vi "Pid_v21.vi"() -> ()   [LabVIEW 2020]
doc: "This example demonstrates how to simulate a general PID controller."
uses:
  <vilib>/addons/control/pid/pid.llb/PID (DBL).vi
  <vilib>/addons/control/pid/NI_PID_pid.lvlib
panel:
  in  "r - Set point":dbl(slide)=4.965034965034965 scale=0.0..10.0
  out "y - Iesirea":dbl(slide)=0.4195804195804196 scale=0.0..10.0
  out "u":dbl(slide)=0.27972027972027974 scale=0.0..10.0
  out "U - comanda":dbl(graph)=4.96503496506626
  in  "PID gains":T1={"proportional gain (Kc)"=20.0, "integral time (Ti, min)"=0.008, "derivative time (Td, min)"=0.001} {"derivative time (Td, min)" format="%.3f"; "integral time (Ti, min)" format="%.3f"; "proportional gain (Kc)" format="%.3f"}
  in  "Stop":bool
  out "u,y,r":T2(graph)={"Plant Output"=4.96503496506626, "output"=4.965034965036714, "r - Set point"=4.965034965034965}
  # "Overview: This example demonstrates how to simulate a simple PID loop controller.\nInstructions:\n1. Run the VI and observe the Process variable (PV) following the Setpoint (SP) value while the output of the controller, also called Manipulated variable (MV), changes to keep both values near each other.\n2. After it settles down (value of PV and SP are near each other), change SP. You can just move the 'blue' arrow on the indicator. The MV will change to drive PV to SP again.\n3. Click Stop to stop the VI."
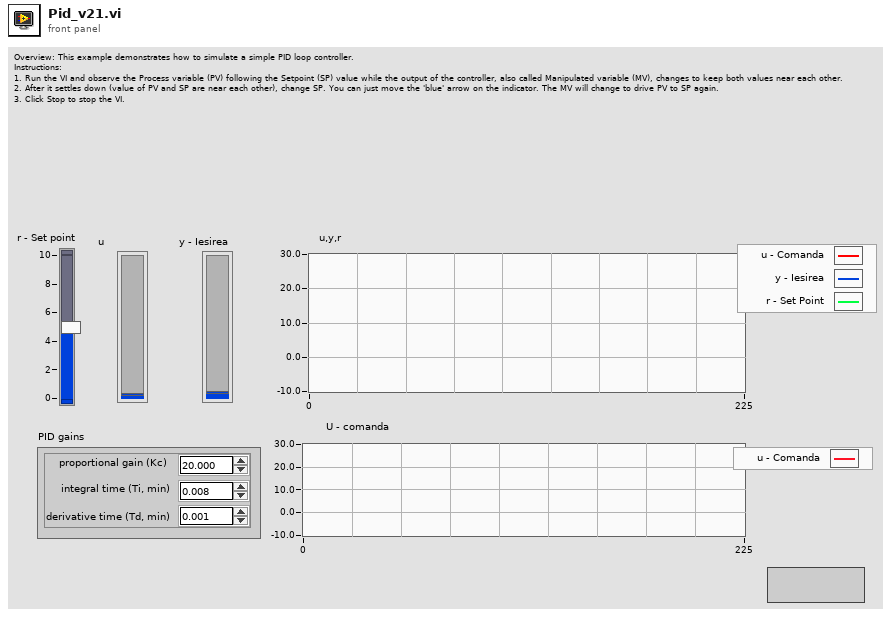
[diagram p1: front panel]
types:
  T1 = cluster{"proportional gain (Kc)":dbl, "integral time (Ti, min)":dbl, "derivative time (Td, min)":dbl}
  T2 = cluster{"Plant Output":dbl, "output":dbl, "r - Set point":dbl}
  T3 = cluster{"output":dbl, "y":dbl, "r - Set point":dbl}
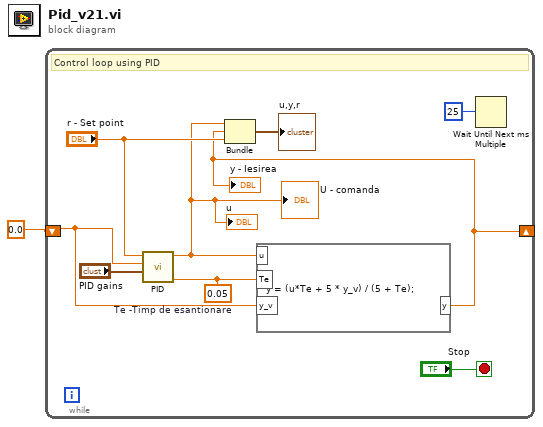
[diagram p0: block diagram]
diagram:
  n1 = while {
    shift-left: 0.0 ("Plant Output") -> [w5]
    shift-right: [w2] -> _
    stop <- "Stop" stop-if-true
    w4 = 0.05  # Te -Timp de esantionare
    # "Control loop using PID"
    n2 = call-poly <vilib>:"PID.vi"("dt (s)"=w4, "PID gains"="PID gains", "process variable"=w5, "setpoint"="r - Set point") -> ("output"=w3:dbl)  [unwired: 6 in, 1 out]
    "U - comanda" <- w3
    "u" <- w3
    n3 = formula code="y = (u*Te + 5 * y_v) / (5 + Te);"("y_v"=w5, "u"=w3, "Te"=w4) -> ("y"=w2:dbl)
    "y - Iesirea" <- w2
    n4 = Bundle("output"=w3, "y"=w2, "r - Set point"="r - Set point") -> (→"u,y,r":T3)  [unwired: 1 in]
    n5 = Wait Until Next ms Multiple(millisecond multiple=u32 25 ("unsigned 32bit integer")) -> ()  [unwired: 1 out]
  }
